vi "Open.vi"(8 "error in (no error)":errorcluster, 11 "Fact in":refnum<class "Fact.lvclass">) -> (0 "error out":errorcluster, 3 "Fact out":refnum<class "Fact.lvclass">)   [LabVIEW 2017, in "Fact.lvclass"]
doc: "Opens the test."
uses:
  Fact.lvclass
  Fact.lvclass/Fact.ctl
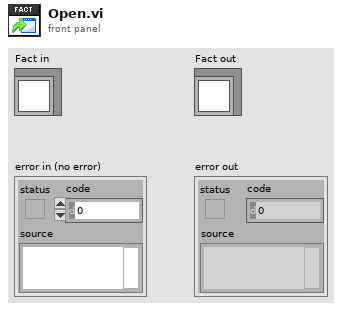
[diagram p1: front panel]
types:
  T1 = enum32{"Invalid", "Standard", "Closed", "Hidden", "Minimized", "Maximized"}
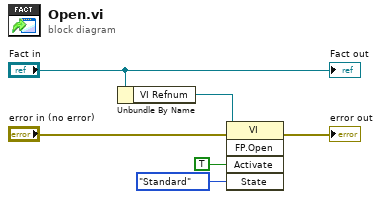
[diagram p0: block diagram]
diagram:
  n1 = Unbundle By Name("Fact in") -> ("VI Refnum"=w3:refnum<vi>)
  n2 = invoke class="VI" method="FP.Open"(reference=w3, error in="error in (no error)", "Activate"=TRUE ("Activate?"), "State"=T1."Standard") -> (error out=→"error out":errorcluster)  [unwired: 1 in, 4 out]
  "Fact out" <- "Fact in"
